vi "Get Package ID.vi"(11 "Test Run Request":refnum<class "Test Run Request.lvclass">) -> (3 "Package ID":string)   [LabVIEW 2026, in "Test Run Request.lvclass"]
uses:
  Test Run Request.lvclass
  Test Run Request.lvclass/Test Run Request.ctl
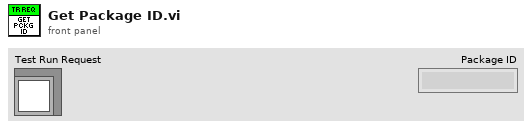
[diagram p1: front panel]
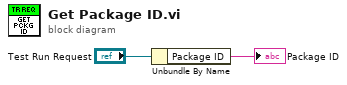
[diagram p0: block diagram]
diagram:
  n1 = Unbundle By Name("Test Run Request") -> ("Package ID"=→"Package ID":string)
